vi "Generate Inlined Image.vi"(8 "error in":errorcluster, 9 "empty":T1, 10 "Name":string, 11 "Image Folder Path":path) -> (0 "error out":errorcluster, 2 "Image String":string, 3 "Image":refnum<class "Image.lvclass">)   [LabVIEW 2021, in "TAF Proj Document Type.lvlib" / "Vi.lvclass"]
uses:
  <vilib>/Wovalab/AntiDoc/Document Type/Add-ons/LabVIEW TAF Project/Vi/Vi.lvclass
  <vilib>/picture/picture.llb/imagedata.ctl
  <vilib>/Wovalab/Asciidoc for LabVIEW/Image/Image.lvclass
  <vilib>/Wovalab/AntiDoc/Document Type/Add-ons/LabVIEW TAF Project/TAF Proj Document Type.lvlib
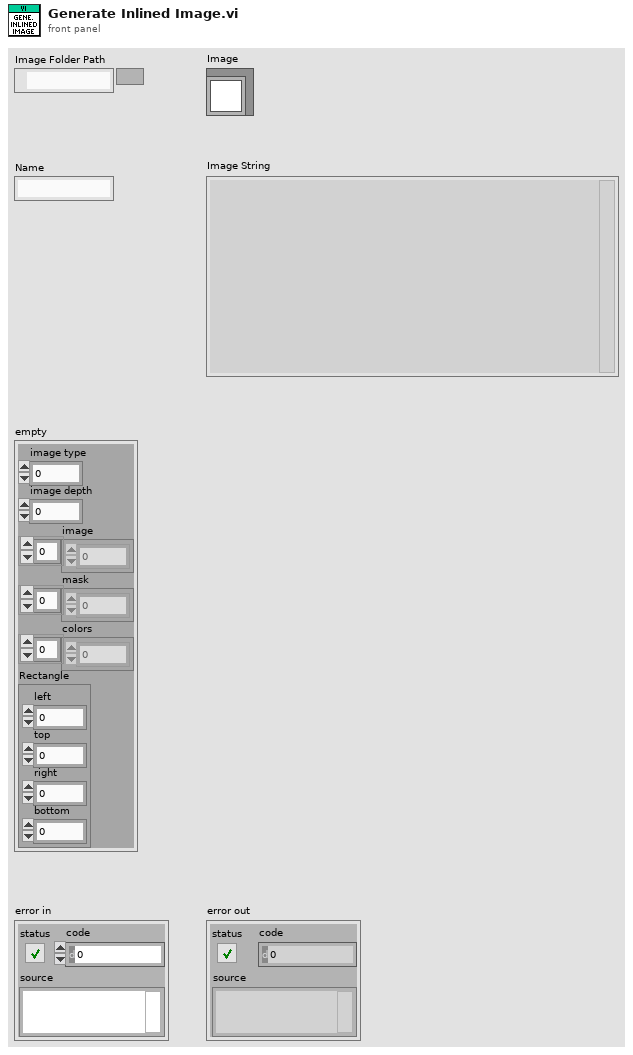
[diagram p1: front panel]
types:
  T1 = typedef "imagedata.ctl" = cluster{"image type":i32, "image depth":i32, "image":u8[], "mask":u8[], "colors":u32[], "Rectangle":cluster{"left":i16, "top":i16, "right":i16, "bottom":i16}}
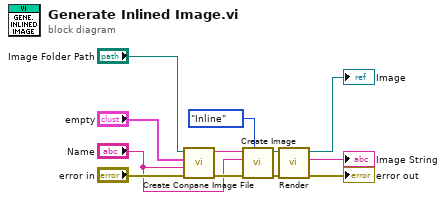
[diagram p0: block diagram]
diagram:
  n1 = call <vilib>:"Create Conpane Image File.vi"("error in"="error in", "Name"="Name", "Conpane Image"="empty", "Image Folder Path"="Image Folder Path") -> ("error out"=w12:errorcluster, "File Name"=w6:string)  [unwired: 6 in]
  n2 = call <vilib>:"Create Image.vi"("Type"=enum16{"Block", "Inline"}."Inline", "error in (no error)"=w12, "Alt Text"="Name", "Image Path"=w6) -> ("error out"=w11:errorcluster, "Image out"=w7:refnum<class "Image.lvclass">)  [unwired: 6 in]
  n3 = call-dynamic "Render.vi"("error in (no error)"=w11, "Adoc-Image in"=w7) -> ("error out"=→"error out":errorcluster, "Output"=→"Image String":string, "Adoc-Image out"=→"Image":refnum<class "Image.lvclass">)  [unwired: 7 in]
